vi "_PC_Daemon_MSConf_SetCtrlState.vi"(6 "exe param memory":T1, 8 "error in (no error)":errorcluster, 11 "Execution.Param":T2={"Method"=path "", "Loops"=1, "AVG"=1, "ContinuesRun"=FALSE}) -> (0 "error out":errorcluster)   [LabVIEW 2018]
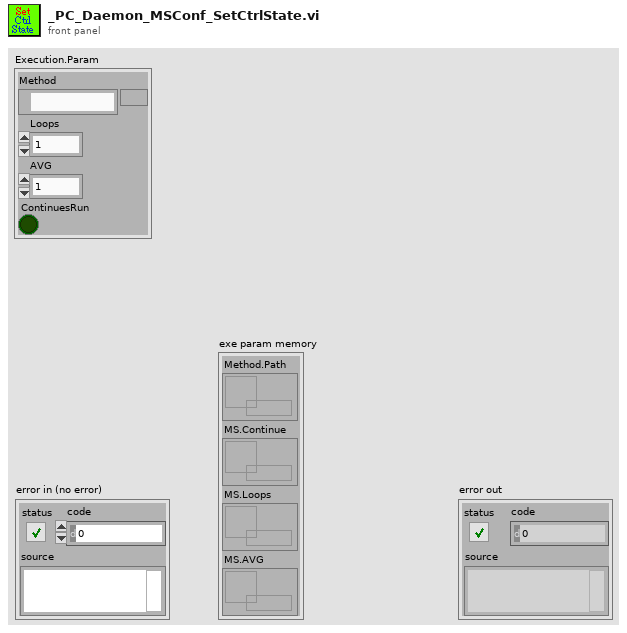
[diagram p1: front panel]
types:
  T1 = cluster{"Method.Path":refnum<data-value>, "MS.Continue":refnum<data-value>, "MS.Loops":refnum<data-value>, "MS.AVG":refnum<data-value>}
  T2 = cluster{"Method":path, "Loops":i32, "AVG":u8, "ContinuesRun":bool}
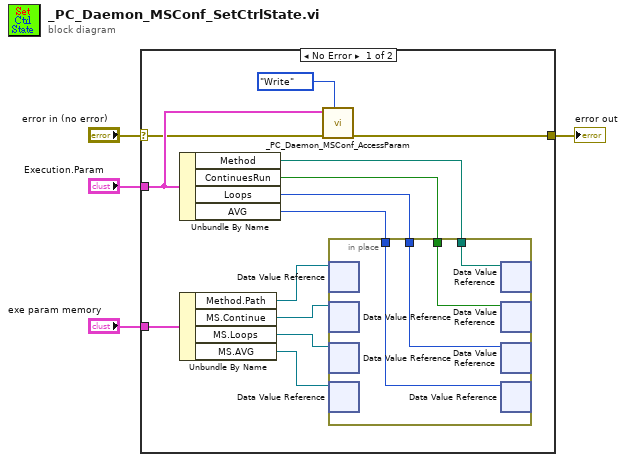
[diagram p0: block diagram]
diagram:
  n1 = case shown="No Error" "error in (no error)" {
    selector: "error in (no error)" -> [w6 w22]
    tunnel: [w5 w22] -> w3
    tunnel: "exe param memory" -> [w13 _]
    tunnel: "Execution.Param" -> [w7 _]
    frame No Error {
      n2 = Unbundle By Name(w7) -> ("Method"=w12:path, "ContinuesRun"=w14:bool, "Loops"=w11:i32, "AVG"=w9:u8)
      n3 = Unbundle By Name(w13) -> ("Method.Path"=w10:refnum<data-value>, "MS.Continue"=w17:refnum<data-value>, "MS.Loops"=w16:refnum<data-value>, "MS.AVG"=w15:refnum<data-value>)
      n4 = call "_PC_Daemon_MSConf_AccessParam.vi"("Function"=enum16{"Write", "Read"}."Write", "error in (no error)"=w6, "Execution.Param in"=w7) -> ("error out"=w5:errorcluster)  [unwired: 7 in, 1 out]
      n5 = in-place {
        in-place-border: w14 -> [w21]
        in-place-border: w12 -> [w20]
        in-place-border: w11 -> [w18]
        in-place-border: w9 -> [w19]
        n6 = in-place-dvr #1(w10) -> ()  [unwired: 2 out]
        n7 = in-place-dvr #2(w17) -> ()  [unwired: 2 out]
        n8 = in-place-dvr #3(w16) -> ()  [unwired: 2 out]
        n9 = in-place-dvr #4(w15) -> ()  [unwired: 2 out]
        n10 = in-place-dvr #1(w20) -> ()  [unwired: 2 out]
        n11 = in-place-dvr #2(w21) -> ()  [unwired: 2 out]
        n12 = in-place-dvr #3(w18) -> ()  [unwired: 2 out]
        n13 = in-place-dvr #4(w19) -> ()  [unwired: 2 out]
      }
    }
    frame Error {
    }
  }
  "error out" <- w3
